vi "Test DMM Card In Slot.vi"(8 "error in (no error)":errorcluster) -> (0 "error out":errorcluster, 2 "In Card Flag":bool)   [LabVIEW 2016, in "Hall Effect Library.lvlib"]
uses:
  Hall Effect Library.lvlib
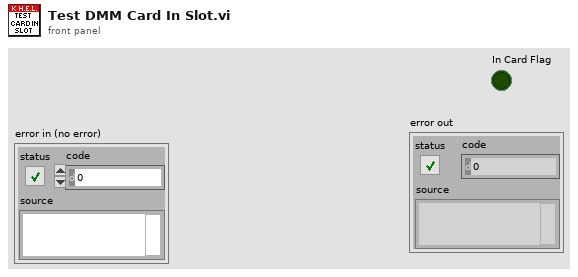
[diagram p1: front panel]
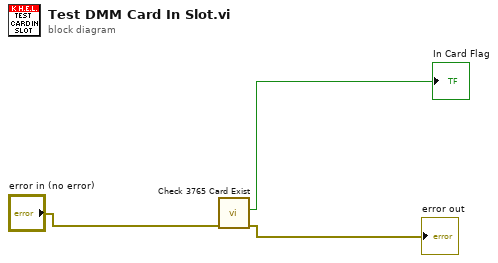
[diagram p0: block diagram]
diagram:
  n1 = call "Check 3765 Card Exist.vi"("error in (no error)"="error in (no error)") -> ("error out"=→"error out":errorcluster, "Boolean"=→"In Card Flag":bool)  [unwired: 9 in]
